vi "U6 Low Latency Stream.vi"() -> ()   [LabVIEW 2021]
panel:
  in  "Delay [ms]":u32
  out "Comm Backlog [%]":dbl format="%.2f"
  in  "Scans To Read Per Iteration":dbl=1.0 format="%.3f"
  out "UD Backlog [%]":dbl format="%.2f"
  out "Actual Scan Rate (Hz)":dbl format="%.3f"
  out "# Scans Read":i32
  out "# of iterations":i32
  out "Data":dbl[][](array[numeric]) format="%.3f"
  in  "Scan Rate (Hz)":dbl=10.0 format="%.3f"
  in  "stop":bool
  out "Error Message":string
  # "Usually command/response is used in low-latency applications.  Stream is good at collecting data fast at precise intervals,\nbut is most efficient when it moves large chunks of data at a time.  This VI demonstrates techniques for moving small\nchunks of data more often."
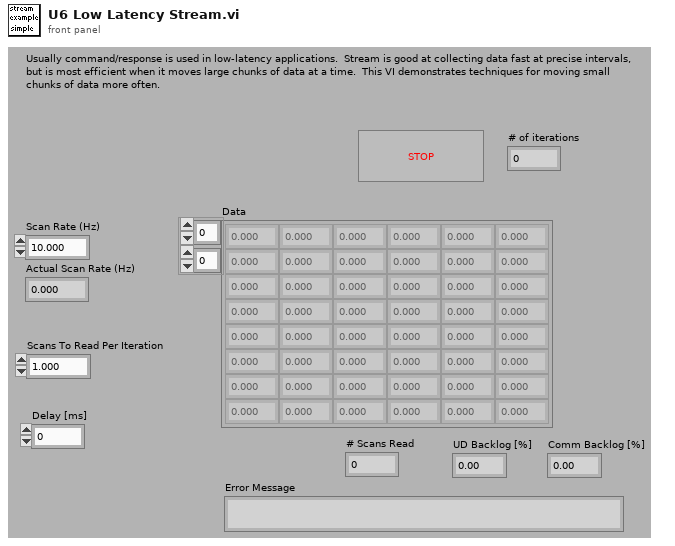
[diagram p1: front panel]
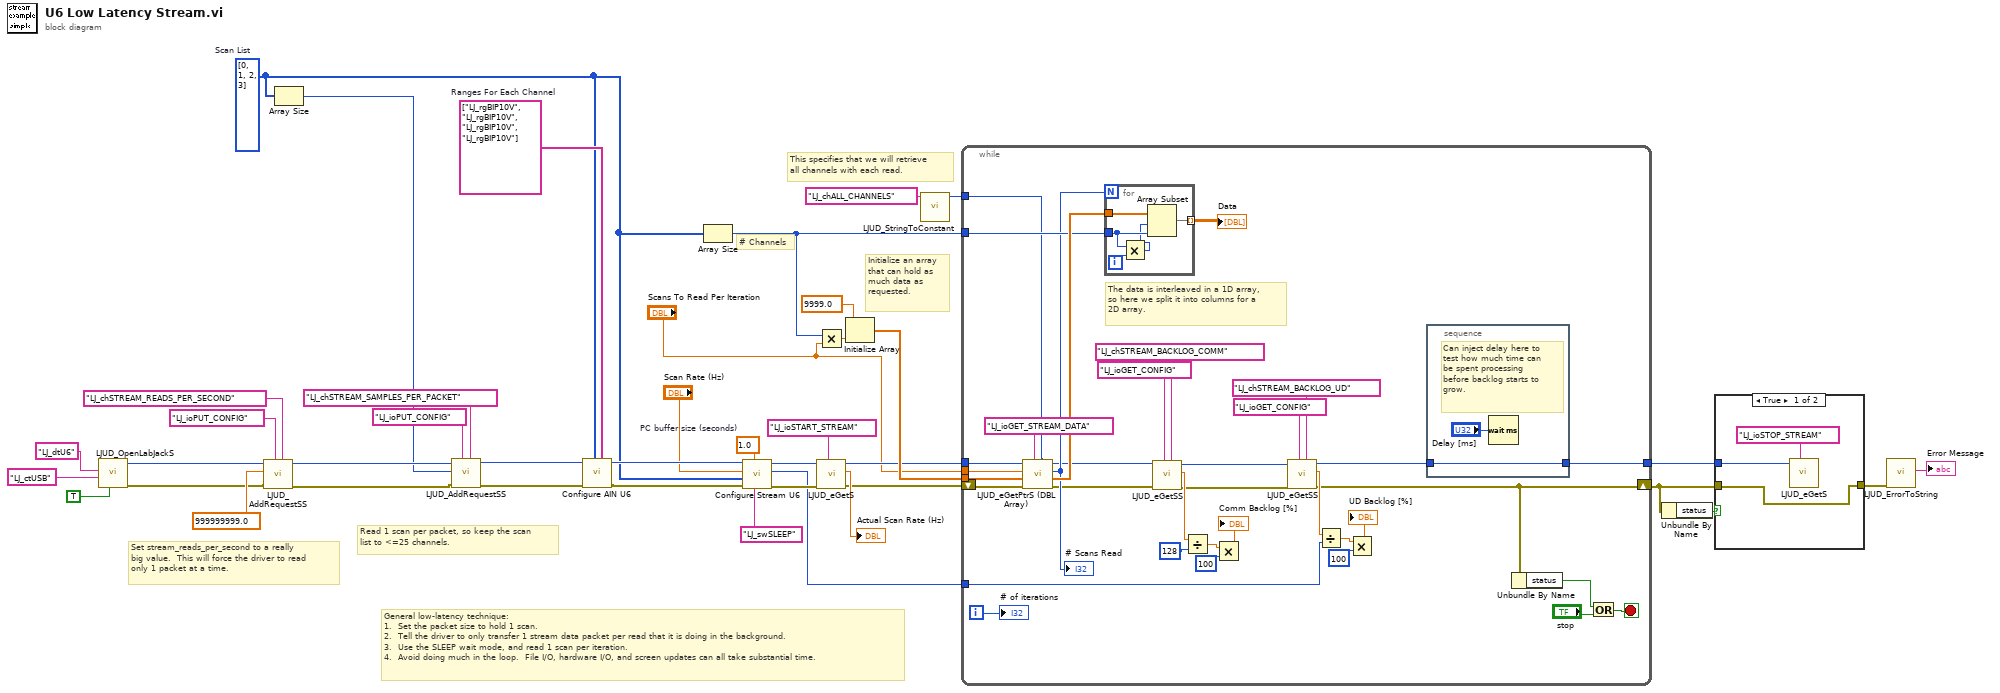
[diagram p0: block diagram]
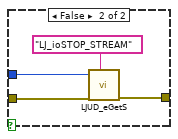
[diagram p2: hidden frame]
diagram:
  w1 = 1.0  # PC buffer size (seconds)
  w4 = i32[] [0, 1, 2, 3]  # Scan List
  w23 = string[] ["LJ_rgBIP10V", "LJ_rgBIP10V", "LJ_rgBIP10V", "LJ_rgBIP10V"]  # Ranges For Each Channel
  # "General low-latency technique:\n1.  Set the packet size to hold 1 scan.\n2.  Tell the driver to only transfer 1 stream data packet per read that it is doing in the background.\n3.  Use the SLEEP wait mode, and read 1 scan per iteration.\n4.  Avoid doing much in the loop.  File I/O, hardware I/O, and screen updates can all take substantial time."
  # "Set stream_reads_per_second to a really\nbig value.  This will force the driver to read\nonly 1 packet at a time."
  # "Read 1 scan per packet, so keep the scan\nlist to <=25 channels."
  # "Initialize an array\nthat can hold as\nmuch data as\nrequested."
  # "# Channels"
  # "This specifies that we will retrieve\nall channels with each read."
  n1 = call "LJUD_OpenLabJackS.vi"("FirstFound"=TRUE, "ConnectionType"="LJ_ctUSB", "DeviceType"="LJ_dtU6") -> ("error out"=w6:errorcluster, "Handle"=w8:i32)  [unwired: 6 in, 1 out]
  n2 = call "LJUD_AddRequestSS.vi"("Channel"="LJ_chSTREAM_READS_PER_SECOND" ("IOType"), "IOType"="LJ_ioPUT_CONFIG", "error in"=w6, "Value"=999999999.0, "Handle In"=w8) -> ("error out"=w5:errorcluster, "Handle Out"=w7:i32)  [unwired: 5 in]
  n3 = Array Size(array=w4) -> (size(s)=w3:i32)
  n4 = call "LJUD_AddRequestSS.vi"("Channel"="LJ_chSTREAM_SAMPLES_PER_PACKET" ("IOType"), "IOType"="LJ_ioPUT_CONFIG", "error in"=w5, "Value"=w3, "Handle In"=w7) -> ("error out"=w18:errorcluster, "Handle Out"=w17:i32)  [unwired: 5 in]
  n5 = call "Configure AIN U6.vi"("Ranges"=w23, "Positive Channels"=w4, "error in"=w18, "Handle In"=w17) -> ("error out"=w29:errorcluster, "Handle Out"=w28:i32)  [unwired: 6 in]
  n6 = Array Size(array=w4) -> (size(s)=w35:i32)
  n7 = call "Configure Stream U6.vi"("Wait Mode"="LJ_swSLEEP" ("Wait Mode (2)"), "PC buffer size (seconds)"=w1, "error in"=w29, "Scan List (+)"=w4, "Scan Rate (Hz)"="Scan Rate (Hz)", "Handle In"=w28) -> ("error out"=w39:errorcluster, "PC buffer size (samples)"=w16:i32, "Handle Out"=w40:i32)  [unwired: 3 in]
  n8 = Multiply(x=w35, y="Scans To Read Per Iteration") -> (x*y=w38:dbl)
  n9 = call "LJUD_eGetS.vi"("IOType"="LJ_ioSTART_STREAM", "error in"=w39, "Handle In"=w40) -> ("error out"=w21:errorcluster, "Value Read"=→"Actual Scan Rate (Hz)":dbl, "Handle Out"=w27:i32)  [unwired: 6 in]
  n10 = Initialize Array(9999.0, w38) -> (w36:dbl[])
  n11 = call "LJUD_StringToConstant.vi"("String"="LJ_chALL_CHANNELS") -> ("Constant Number"=w24:i32)  [unwired: 9 in, 1 out]
  n12 = while {
    tunnel: w16 -> [w55]
    shift-left: w21 -> [w63]
    shift-right: [w56] -> w22
    tunnel: w24 -> [w66]
    tunnel: [w53] -> w33
    tunnel: w35 -> [w69]
    tunnel: w36 -> [w72]
    tunnel: "Scans To Read Per Iteration" -> [w70]
    tunnel: w27 -> [w74]
    i -> [w68]
    stop <- w65 stop-if-true
    # "The data is interleaved in a 1D array,\nso here we split it into columns for a\n2D array."
    n13 = call "LJUD_eGetPtrS (DBL Array).vi"("Channel"=w66, "IOType"="LJ_ioGET_STREAM_DATA", "error in"=w63, "DBL Array Write"=w72, "Value"=w70, "Handle In"=w74) -> ("error out"=w44:errorcluster, "DBL Array Read"=w71:dbl[], "Value"=w64:i32, "Handle Out"=w43:i32)  [unwired: 2 in]
    "# Scans Read" <- w64
    n14 = for {
      N: w64 -> [_]
      tunnel: w71 -> [w83]
      tunnel: w69 -> [w82]
      tunnel: [w79] -> w67 mode=indexing
      i -> [w81]
      n15 = Multiply(x=w82, y=w81) -> (x*y=w80:i32)
      n16 = Array Subset(array=w83, index=w80, length=w82) -> (w79:dbl[])
    }
    "Data" <- w67
    n17 = call "LJUD_eGetSS.vi"("Channel"="LJ_chSTREAM_BACKLOG_COMM", "IOType"="LJ_ioGET_CONFIG", "error in"=w44, "Handle In"=w43) -> ("error out"=w45:errorcluster, "Value Read"=w52:dbl, "Handle Out"=w46:i32)  [unwired: 5 in]
    n18 = Divide(x=w52, y=128) -> (x/y=w49:dbl)
    n19 = Multiply(x=w49, y=100) -> (x*y=→"Comm Backlog [%]":dbl)
    n20 = call "LJUD_eGetSS.vi"("Channel"="LJ_chSTREAM_BACKLOG_UD", "IOType"="LJ_ioGET_CONFIG", "error in"=w45, "Handle In"=w46) -> ("error out"=w56:errorcluster, "Value Read"=w58:dbl, "Handle Out"=w54:i32)  [unwired: 5 in]
    n21 = Divide(x=w58, y=w55) -> (x/y=w59:dbl)
    n22 = Multiply(x=w59, y=100) -> (x*y=→"UD Backlog [%]":dbl)
    n23 = stacked-sequence {
      tunnel: w54 -> [w78]
      tunnel: [w78] -> w53
      frame #0 {
        # "Can inject delay here to\ntest how much time can\nbe spent processing\nbefore backlog starts to\ngrow."
        n24 = Wait (ms)(milliseconds to wait="Delay [ms]") -> ()  [unwired: 1 out]
      }
    }
    n25 = Unbundle By Name(w56) -> ("status"=w75:bool)
    n26 = Or(x=w75, y="stop") -> (x .or. y?=w65:bool)
    "# of iterations" <- w68
  }
  n27 = Unbundle By Name(w22) -> ("status"=w26:bool)
  n28 = case shown="True" w26 {
    tunnel: w33 -> [w85 w89]
    tunnel: [w84 w88] -> w32
    tunnel: w22 -> [w84 w87]
    frame True {
      n29 = call "LJUD_eGetS.vi"("IOType"="LJ_ioSTOP_STREAM", "Handle In"=w85) -> ()  [unwired: 7 in, 3 out]
    }
    frame False {
      n30 = call "LJUD_eGetS.vi"("IOType"="LJ_ioSTOP_STREAM", "error in"=w87, "Handle In"=w89) -> ("error out"=w88:errorcluster)  [unwired: 6 in, 2 out]
    }
  }
  n31 = call "LJUD_ErrorToString.vi"("error in"=w32) -> ("String"=→"Error Message":string)  [unwired: 10 in]
